vi "Untitled 2.vi"(8 "error in (no error)":errorcluster, 11 "USB-6000 in":refnum<class "USB-6000.lvclass">) -> (0 "error out":errorcluster, 3 "USB-6000 out":refnum<class "USB-6000.lvclass">)   [LabVIEW 2025, in "USB IO.lvlib" / "USB-6000.lvclass"]
uses:
  USB-6000.lvclass
  USB-6000.lvclass/USB-6000.ctl
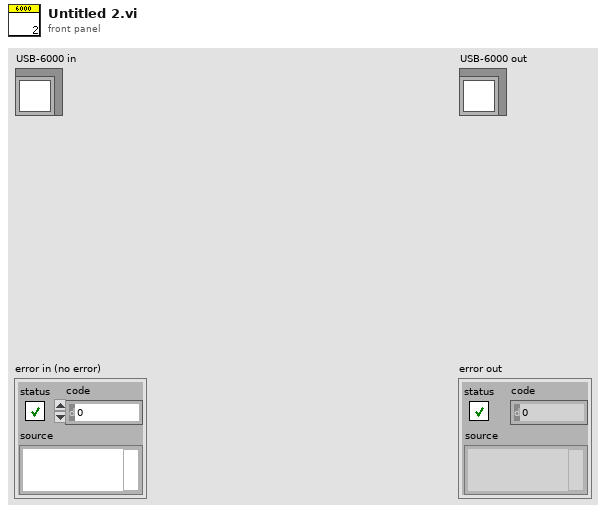
[diagram p1: front panel]
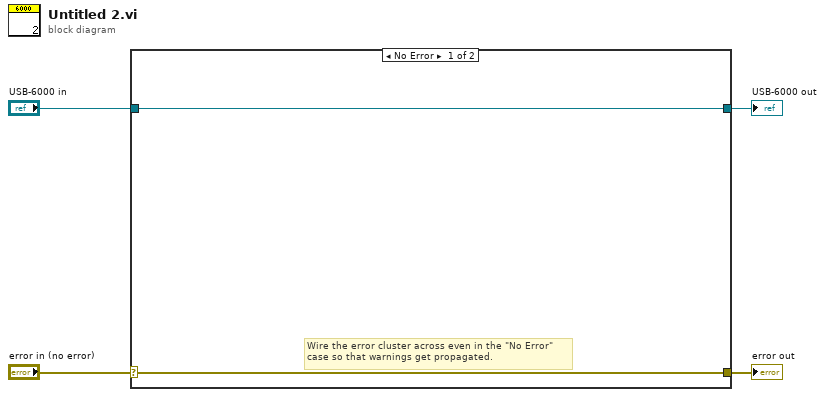
[diagram p0: block diagram]
diagram:
  n1 = case shown="No Error" "error in (no error)" {
    selector: "error in (no error)" -> [w5 w8]
    tunnel: [w5 w8] -> w3
    tunnel: [w6 w7] -> w1
    tunnel: "USB-6000 in" -> [w6 w7]
    frame No Error {
      # "Wire the error cluster across even in the \"No Error\"\ncase so that warnings get propagated."
    }
    frame Error {
    }
  }
  "error out" <- w3
  "USB-6000 out" <- w1
